vi "Spartan HTTP Build Header.vi"(8 "add separator (T)":bool=TRUE, 9 "content length (-1)":i32=-1, 10 "server-push header (F)":bool, 11 "header":string) -> (1 "status":i32, 2 "content-type":string, 3 "full header":string)   [LabVIEW 2011]
uses:
  ITK EXT/utils/keyedarr.llb/Keyed Array.ctl
panel:
  out "full header":bool
  in  "default header":T1
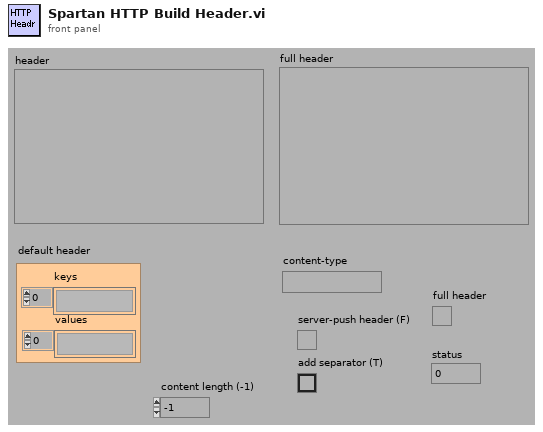
[diagram p1: front panel]
types:
  T1 = typedef "Keyed Array.ctl" = cluster{"keys":string[], "values":string[]}
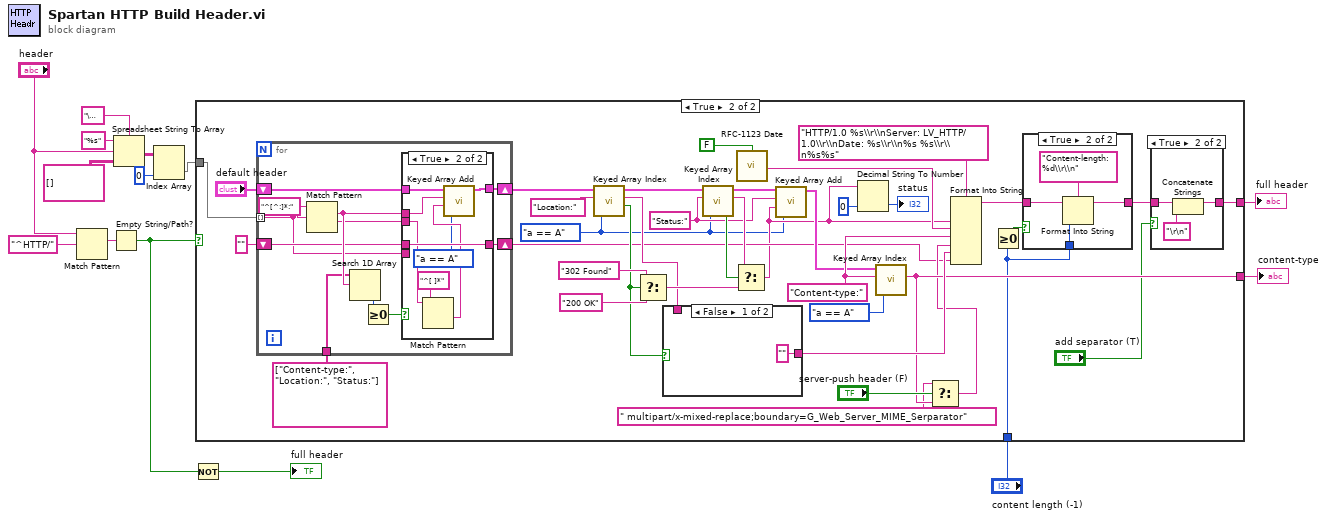
[diagram p0: block diagram]
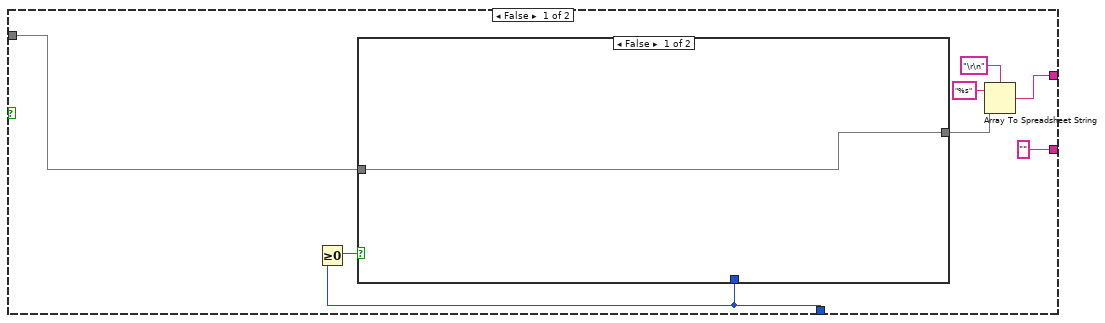
[diagram p2: hidden frame]
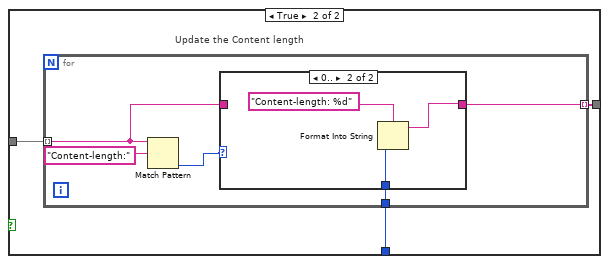
[diagram p3: hidden frame]
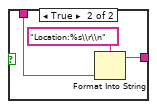
[diagram p7: hidden frame]
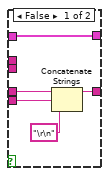
[diagram p8: hidden frame]
diagram:
  n1 = Match Pattern(string="header", regular expression="^HTTP/") -> (match substring=w13:string)  [unwired: 4 out]
  n2 = Empty String/Path?(string/path=w13) -> (empty?=w2:bool)
  n3 = Spreadsheet String To Array(delimiter (Tab)="\u0000" ("format string"), format string="%s", spreadsheet string="header", array type (2D Dbl)=string[][] []) -> (array=w9:string[][])
  n4 = Index Array(array=w9, index (col)=0) -> (element=w7:string[])  [unwired: 1 in]
  n5 = Not(x=w2) -> (.not. x?=→"full header":bool)
  n6 = case shown="True" w2 {
    tunnel: w7 -> [w18 w71]
    tunnel: [w20 w45] -> w5
    tunnel: ["" ("value") w55] -> w4
    tunnel: "content length (-1)" -> [w16 w36]
    frame False {
      n7 = Greater Or Equal To 0?(x=w16) -> (x >= 0?=w15:bool)
      n8 = case shown="False" w15 {
        tunnel: w18 -> [w23 w26]
        tunnel: [w23 w25] -> w17
        tunnel: w16 -> [_ w24]
        frame False {
        }
        frame True {
          # "Update the Content length"
          n9 = for {
            tunnel: w26 -> [w29] mode=indexing
            tunnel: [w28] -> w25 mode=indexing
            tunnel: w24 -> [w27]
            n10 = Match Pattern(string=w29, regular expression="Content-length:" ("format string")) -> (offset past match=w30:i32)  [unwired: 4 out]
            n11 = case shown="0.." w30 {
              tunnel: [w32 w33] -> w28
              tunnel: w29 -> [w32 _]
              tunnel: w27 -> [_ w34]
              frame Default {
              }
              frame 0.. {
                n12 = Format Into String(format string="Content-length: %d", w34) -> (resulting string=w33:string)  [unwired: 2 in, 1 out]
              }
            }
          }
        }
      }
      n13 = Array To Spreadsheet String(delimiter (Tab)="\r\n", array=w17, 3:"%s" ("format string")) -> (spreadsheet string=w20:string)
    }
    frame True {
      w37 = enum16{"a != A", "a == A", "system"}."a == A" ("case matching (sensitive)")
      w61 = "Content-type:"
      w50 = "Status:" ("key")
      n14 = for {
        tunnel: w71 -> [w86] mode=indexing
        shift-right: [w89] -> w68
        shift-left: "default header" -> [w90]
        tunnel: string[] ["Content-type:", "Location:", "Status:"] -> [w88]
        shift-right: [w85] -> w42
        shift-left: "" -> [w87]
        n15 = Match Pattern(string=w86, regular expression="^[^:]*:") -> (match substring=w92:string, after substring=w91:string)  [unwired: 3 out]
        n16 = Search 1D Array(1D array=w88, element=w92) -> (index of element=w94:i32)  [unwired: 1 out]
        n17 = Greater Or Equal To 0?(x=w94) -> (x >= 0?=w93:bool)
        n18 = case shown="True" w93 {
          tunnel: w92 -> [_ w107]
          tunnel: w91 -> [_ w104]
          tunnel: w90 -> [w100 w108]
          tunnel: [w100 w106] -> w89
          tunnel: w87 -> [w99 w105]
          tunnel: w86 -> [w98 _]
          tunnel: [w97 w105] -> w85
          frame False {
            n19 = Concatenate Strings(w99, w98, "\r\n" ("key")) -> (w97:string)
          }
          frame True {
            n20 = Match Pattern(string=w104, regular expression="^[ ]*") -> (after substring=w103:string)  [unwired: 4 out]
            n21 = call "Keyed Array Add.vi"("case matching (sensitive)"=enum16{"a != A", "a == A", "system"}."a == A", "value"=w103, "key"=w107, "array in"=w108) -> ("array out"=w106:T1)  [unwired: 3 out]
          }
        }
      }
      n22 = call "Keyed Array Index.vi"("case matching (sensitive)"=w37, "key"="Location:", "array in"=w68) -> ("valid key"=w59:bool, "value"=w58:string)  [unwired: 1 in, 2 out]
      n23 = Select(t="302 Found" ("key"), s=w59, f="200 OK" ("key")) -> (s? t:f=w63:string)
      n24 = case shown="False" w59 {
        tunnel: w58 -> [_ w83]
        tunnel: ["" w82] -> w57
        frame False {
        }
        frame True {
          n25 = Format Into String(format string="Location:%s\\r\\n", w83) -> (resulting string=w82:string)  [unwired: 2 in, 1 out]
        }
      }
      n26 = call "Keyed Array Index.vi"("case matching (sensitive)"=w37, "key"=w50, "array in"=w68) -> ("valid key"=w65:bool, "value"=w64:string)  [unwired: 1 in, 2 out]
      n27 = Select(t=w64, s=w65, f=w63) -> (s? t:f=w41:string)
      n28 = call "RFC-1123 Date.vi"("numeric zone offset (true)"=FALSE) -> ("GMT Date/Time"=w52:string)  [unwired: 1 in]
      n29 = call "Keyed Array Add.vi"("case matching (sensitive)"=w37, "value"=w41, "key"=w50, "array in"=w68) -> ("array out"=w49:T1)  [unwired: 3 out]
      n30 = Decimal String To Number(string=w41, default (0L)=0) -> (number=→"status":i32)  [unwired: 2 out]
      n31 = call "Keyed Array Index.vi"("case matching (sensitive)"=enum16{"a != A", "a == A", "system"}."a == A", "key"=w61, "array in"=w49) -> ("value"=w55:string)  [unwired: 1 in, 3 out]
      n32 = Select(t=" multipart/x-mixed-replace;boundary=G_Web_Server_MIME_Serparator", s="server-push header (F)", f=w55) -> (s? t:f=w54:string)
      n33 = Format Into String(format string="HTTP/1.0 %s\\r\\nServer: LV_HTTP/1.0\\r\\nDate: %s\\r\\n%s %s\\r\\n%s%s", w41, w52, w61, w54, w57, w42) -> (resulting string=w47:string)  [unwired: 2 in, 1 out]
      n34 = Greater Or Equal To 0?(x=w36) -> (x >= 0?=w48:bool)
      n35 = case shown="True" w48 {
        tunnel: w47 -> [w76 w79]
        tunnel: w36 -> [_ w78]
        tunnel: [w76 w77] -> w46
        frame False {
        }
        frame True {
          n36 = Format Into String(format string="Content-length: %d\\r\\n", initial string=w79, w78) -> (resulting string=w77:string)  [unwired: 1 in, 1 out]
        }
      }
      n37 = case shown="True" "add separator (T)" {
        tunnel: w46 -> [w72 w75]
        tunnel: [w72 w74] -> w45
        frame False {
        }
        frame True {
          n38 = Concatenate Strings(w75, "\r\n") -> (w74:string)
        }
      }
    }
  }
  "full header" <- w5
  "content-type" <- w4
